vi "LV86_32 bit array to image.vi"(0 "Intensity Graph":u32[][](graph), 2 "Flip?":bool, 3 "Image In":T1 {"Dialogs" format="%.0b"}) -> (1 "Image Out":T1 {"Dialogs" format="%.0b"})   [LabVIEW 2024]
doc: "This VI converts a 2-dimensional array to a color image. The image resolution is equal to the number of columns by the number of rows. The 32 bits are encoded as first 8 bits are Blue, second 8 bits are Green, third are Red and the last 8 bits are the greyscale.\n\nModifier: \nFlip: If true, this will flip the image so that the image looks right in the Intensity graph (element 0,0 in a picture is the upper left corner but in a graph is in the lower left). Default is False."
uses:
  <userlib>/ImageProcessing/QTLIB_2595_LV86/QT_Image.ctl
panel:
  # "This VI converts a 2-dimensional array to a color image.  The image resolution is equal to the number of columns by the number of rows. The 32 bits are encoded as first 8 bits are Blue, second 8 bits are Green, third are Red and the last 8 bits are the greyscale.\n\nModifier: \nFlip: If true, this will flip the image so that the image looks right in the Intensity graph (element 0,0  in a picture is the upper left corner but in a graph is in the lower left).  Default is False."
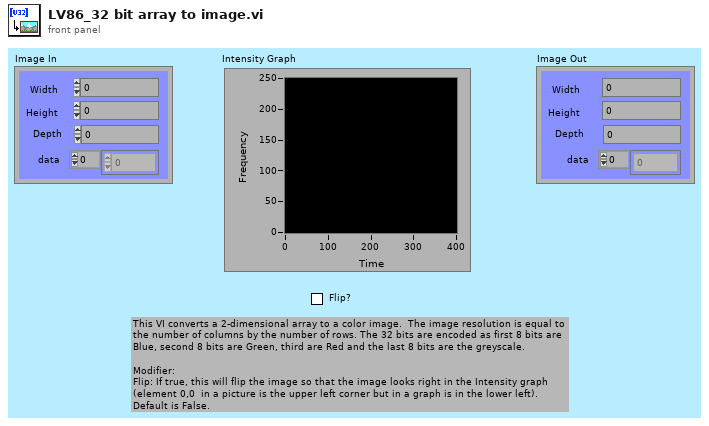
[diagram p1: front panel]
types:
  T1 = typedef "QT_Image.ctl" = cluster{"Width":i32, "Height":i32, "Depth":i32, "data":u8[], "Compressed data":u8[], "Color table":u32[], "Duration":i32, "Options":i32, "Timestamp":i32, "ID":i32, "Reserved":i32, "Dialogs":u32}
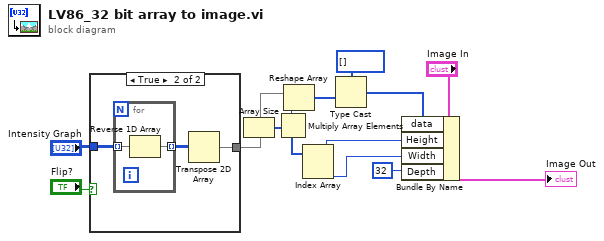
[diagram p0: block diagram]
diagram:
  n1 = case shown="True" "Flip?" {
    tunnel: "Intensity Graph" -> [w14 w17]
    tunnel: [w14 w15] -> w5
    frame False {
    }
    frame True {
      n2 = for {
        tunnel: w17 -> [w19] mode=indexing
        tunnel: [w18] -> w16 mode=indexing
        n3 = Reverse 1D Array(array=w19) -> (reversed array=w18:u32[])
      }
      n4 = Transpose 2D Array(2D array=w16) -> (transposed array=w15:u32[][])
    }
  }
  n5 = Array Size(array=w5) -> (size(s)=w11:i32[])
  n6 = Multiply Array Elements(1:w11) -> (0:w10:i32)
  n7 = Reshape Array(w5, w10) -> (w4:u32[])
  n8 = Index Array(array=w11) -> (element #1=w9:i32, element #2=w8:i32)  [unwired: 2 in]
  n9 = Type Cast(type=u8[] [] ("Array Constant"), x=w4) -> (*(type *) &x=w2:u8[])
  n10 = Bundle By Name(cluster="Image In", "data"=w2, "Height"=w9, "Width"=w8, "Depth"=32) -> (→"Image Out":T1)
